vi "Default FP Window Size - Message Log.vi"() -> (2 "Height":i16=649, 3 "Width":i16=878)   [LabVIEW 2017, in "Settings.lvclass"]
uses:
  Settings.lvclass
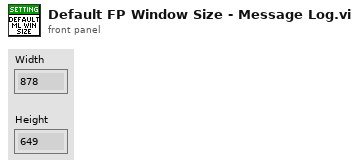
[diagram p1: front panel]
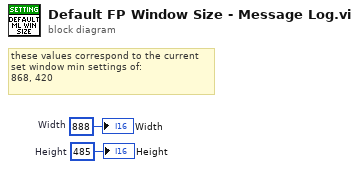
[diagram p0: block diagram]
diagram:
  w2 = i16 485  # Height
  w1 = i16 888  # Width
  # "these values correspond to the current\nset window min settings of:\n868, 420"
  "Height" <- w2
  "Width" <- w1
